vi "MX Component.vi"(8 "错误输入":errorcluster, 10 "Component Assemble Input":T1, 11 "MX操作选项":T3) -> (0 "错误输出":errorcluster, 2 "Component Assemble Output":T1, 3 "State Assemble":T2)   [LabVIEW 2017]
uses:
  Component Assemble Input.ctl
  State Assemble.ctl
panel:
  in  "选项卡控件":enum32{"选项卡 1"}(tab)
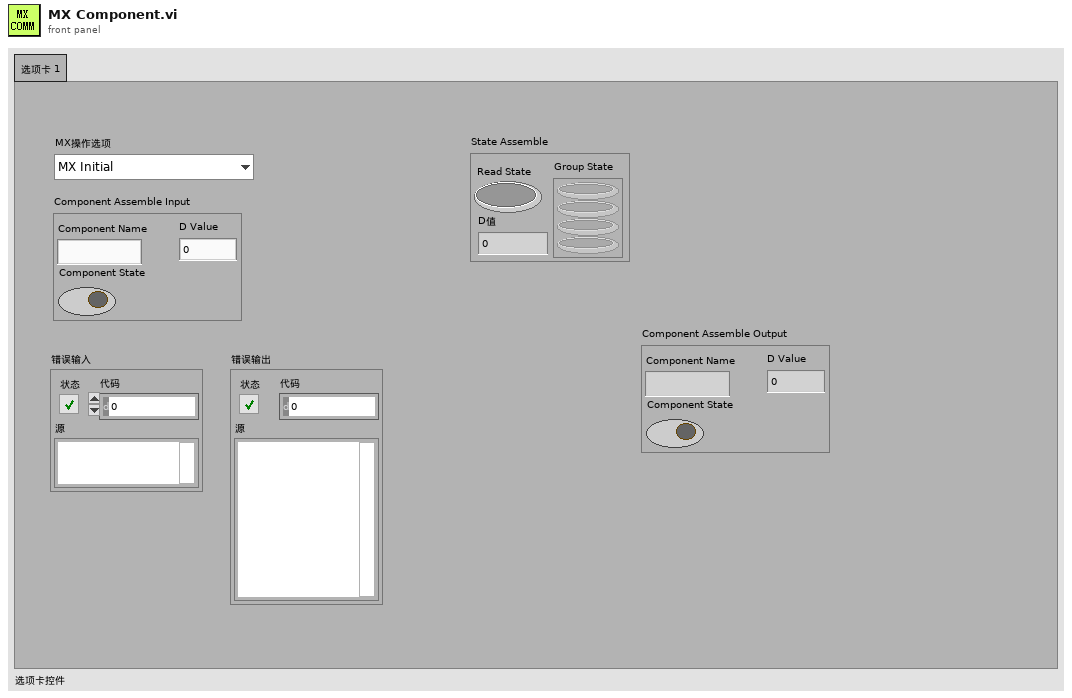
[diagram p1: front panel]
types:
  T1 = typedef "Component Assemble Input.ctl" = cluster{"Component Name":string, "Component State":bool, "D Value":i32}
  T2 = typedef "State Assemble.ctl" = cluster{"Read State":bool, "Group State":bool[], "D值":i32}
  T3 = typedef "MX操作选项.ctl" = enum16{"MX Initial ", "MX Close", "X&Y&M Read", "X&Y&M Write", "D Read", "D Write", "Many component Read", "Many component Write", "Load Function Global"}
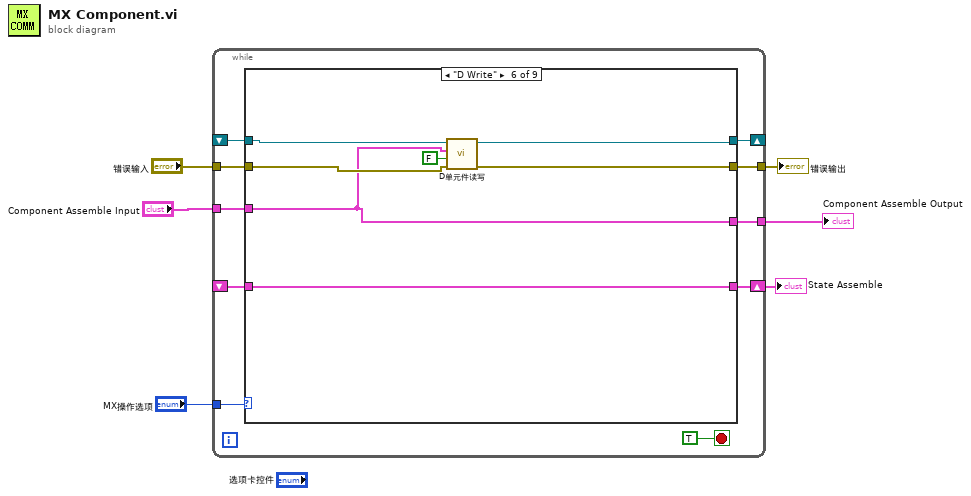
[diagram p0: block diagram]
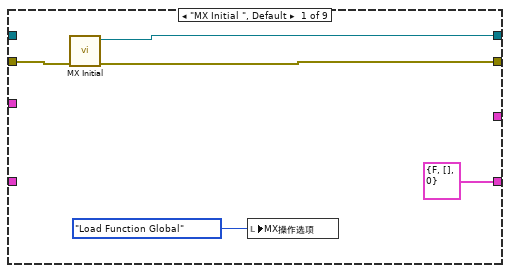
[diagram p2: hidden frame]
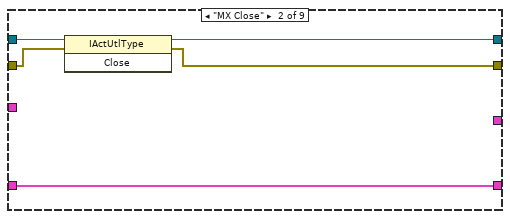
[diagram p3: hidden frame]
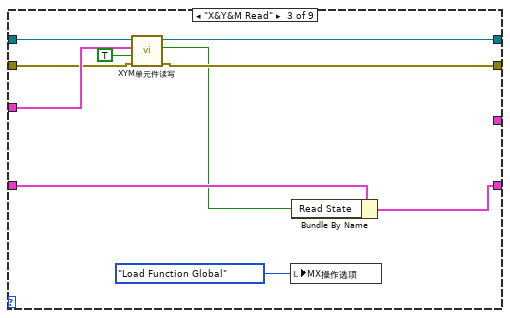
[diagram p4: hidden frame]
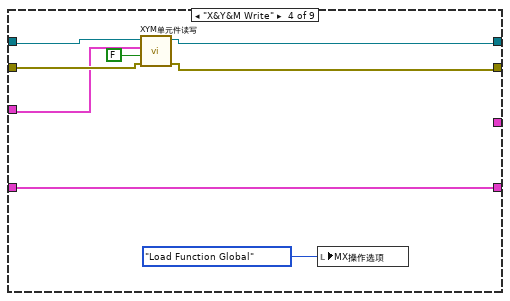
[diagram p5: hidden frame]
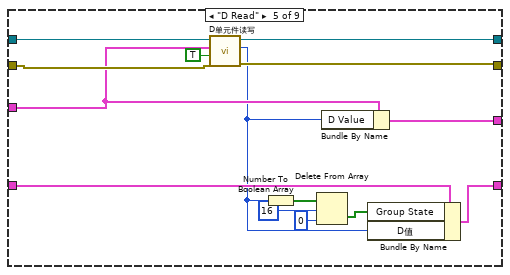
[diagram p6: hidden frame]
diagram:
  n1 = while {
    tunnel: "MX操作选项" -> [w15]
    shift-right: [w13] -> _
    shift-left: _ -> [w11]
    tunnel: "错误输入" -> [w14]
    tunnel: [w12] -> w4
    tunnel: "Component Assemble Input" -> [w10]
    shift-right: [w9] -> w2
    shift-left: _ -> [w8]
    tunnel: [w7] -> w1
    stop <- TRUE stop-if-true
    n2 = case shown="\"D Write\"" w15 {
      tunnel: w14 -> [w21 w25 w33 w42 w57 w63 w67 w70 w73]
      tunnel: [w20 w23 w32 w40 w56 w62 w68 w71 w74] -> w13
      tunnel: [w19 w24 w31 w39 w55 w61 w67 w70 w73] -> w12
      tunnel: w11 -> [_ w26 w36 w43 w58 w64 w68 w71 w74]
      tunnel: w10 -> [_ _ w35 w41 w47 w59 _ _ _]
      tunnel: [T2 {"Read State"=FALSE, "Group State"=[], "D值"=0} ("State Assemble") w22 w28 w38 w52 w60 w66 w69 w72] -> w9
      tunnel: w8 -> [_ w22 w30 w38 w53 w60 w66 w69 w72]
      tunnel: [_ _ _ _ w45 w59 _ _ _] -> w7
      frame "MX Initial ", Default {
        n3 = call "MX Initial.vi"("错误输入"=w21) -> ("错误输出"=w19:errorcluster, "引用输出"=w20:refnum<k7>)  [unwired: 9 in]
        n4 = local write "MX操作选项"(MX操作选项."Load Function Global" ("MX操作选项")) -> ()
      }
      frame "MX Close" {
        n5 = invoke on="调用节点" class="IActUtlType" method="Close"(reference=w26, error in=w25) -> (reference out=w23:refnum<k7>, error out=w24:errorcluster)  [unwired: 1 in, 1 out]
      }
      frame "X&Y&M Read" {
        n6 = call "XYM单元件读写.vi"("错误输入"=w33, "Read？"=TRUE, "Component Assemble Input"=w35, "引用"=w36) -> ("错误输出"=w31:errorcluster, "Read State"=w29:bool, "引用输出"=w32:refnum<k7>)  [unwired: 5 in]
        n7 = local write "MX操作选项"(MX操作选项."Load Function Global" ("MX操作选项")) -> ()
        n8 = Bundle By Name(cluster=w30, "Read State"=w29) -> (w28:T2)
      }
      frame "X&Y&M Write" {
        n9 = call "XYM单元件读写.vi"("错误输入"=w42, "Read？"=FALSE, "Component Assemble Input"=w41, "引用"=w43) -> ("错误输出"=w39:errorcluster, "引用输出"=w40:refnum<k7>)  [unwired: 5 in, 1 out]
        n10 = local write "MX操作选项"(MX操作选项."Load Function Global" ("MX操作选项")) -> ()
      }
      frame "D Read" {
        n11 = call "D单元件读写.vi"("错误输入"=w57, "Read？"=TRUE, "Component Assemble Input"=w47, "引用"=w58) -> ("错误输出"=w55:errorcluster, "D Value"=w46:i32, "引用输出"=w56:refnum<k7>)  [unwired: 5 in]
        n12 = Number To Boolean Array(number=w46) -> (Boolean array=w51:bool[])
        n13 = Delete From Array(array=w51, length=16 ("长度"), index=0 ("索引")) -> (deleted portion=w48:bool[])  [unwired: 1 out]
        n14 = Bundle By Name(cluster=w47, "D Value"=w46) -> (w45:T1)
        n15 = Bundle By Name(cluster=w53, "Group State"=w48, "D值"=w46) -> (w52:T2)
      }
      frame "D Write" {
        n16 = call "D单元件读写.vi"("错误输入"=w63, "Read？"=FALSE, "Component Assemble Input"=w59, "引用"=w64) -> ("错误输出"=w61:errorcluster, "引用输出"=w62:refnum<k7>)  [unwired: 5 in, 1 out]
      }
      frame "Many component Read" {
      }
      frame "Many component Write" {
      }
      frame "Load Function Global" {
      }
    }
  }
  "错误输出" <- w4
  "State Assemble" <- w2
  "Component Assemble Output" <- w1
